vi "ImportCSV.vi"() -> ()   [LabVIEW 2019]
uses:
  System Explorer/RefMem DMA System Explorer.lvlib
panel:
  out "error out":errorcluster
  in  "CSV File Path 2":path
  # "Header\tDefinition\nBlockName\tIt’s the DMA BlockName, same name for all Channels from that given Block.\nBlock Offset (Doubles)\tIt’s the DMA Block Offset (in Doubles), same Offset for all Channels from that Block.\nBlock Direction (Read or Write)\tIt’s either “Read” or “Write”, no other values supported. All Channels from that block must be set to same Direction value.\nChannel Relative Offset (Doubles)\tIt’s the Relative Offset of that Channel within considered DMA Block. For Read Direction, there might be gaps (addresses not used within the Block). For Write Direction all Offsets must be present.\nChannel Name\tNI-VeriStand Channel Name.\nChannel Unit\tUnit for that Channel. It can be omitted (empty string).\nChannel Default Value (for Write Channels Only)\tValue used as Init Value for that NI-VeriStand Channel. Note that it applies only for Write Direction. It can be omitted (empty string)."
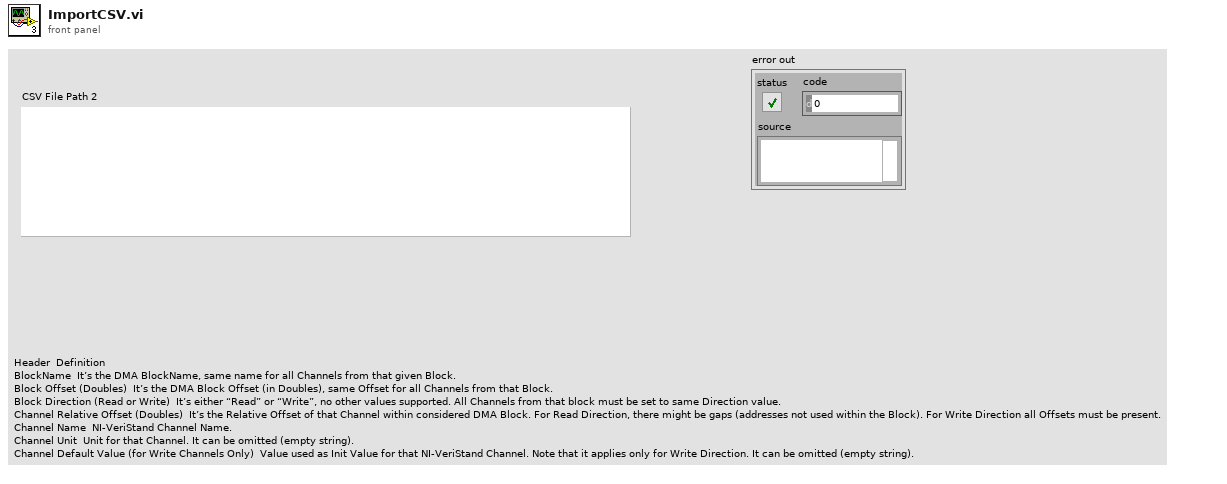
[diagram p1: front panel]
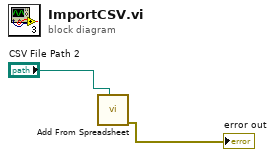
[diagram p0: block diagram]
diagram:
  n1 = call "Add From Spreadsheet.vi"("file path (use dialog)"="CSV File Path 2") -> ("error out"=→"error out":errorcluster)  [unwired: 10 in]
